vi "Parse Cal String.vi"(3 "error in (no error)":errorcluster={"status"=FALSE, "code"=1073676294, "source"="VISA Read in Read Cal Response.vi"}, 5 "read buffer in":string="19:30:28 105, -1, 1.955 1.954 1.95565 1.954") -> (0 "error out":errorcluster={"status"=FALSE, "code"=1073676294, "source"="VISA Read in Read Cal Response.vi"}, 1 "Cal Data":T1={"Time"="19:30:28", "Consecutive good readings"=105, "Total good readings"=-1, "A/D counts Sensor 1"=1.955, "A/D counts Sensor 2"=1.954, "Diff current/previous Sensor 1"=1.95565, "Diff current/previous Sensor 2"=1.954}, 2 "CAL Complete":bool=TRUE)   [LabVIEW 2013]
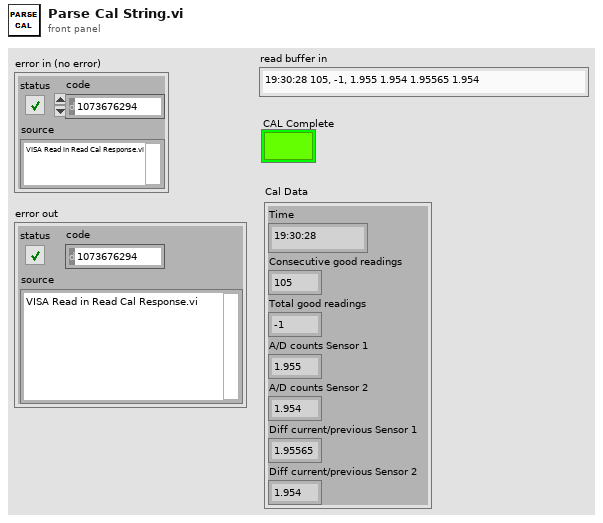
[diagram p1: front panel]
types:
  T1 = cluster{"Time":string, "Consecutive good readings":i32, "Total good readings":i32, "A/D counts Sensor 1":sgl, "A/D counts Sensor 2":sgl, "Diff current/previous Sensor 1":sgl, "Diff current/previous Sensor 2":sgl}
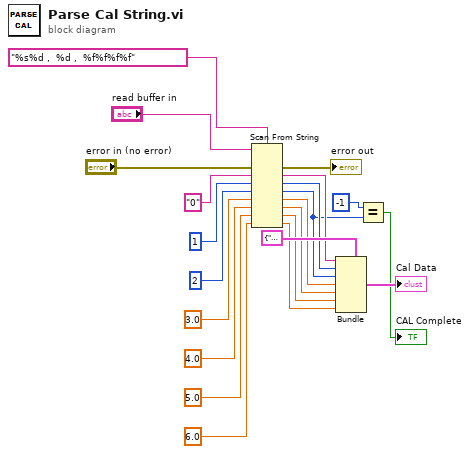
[diagram p0: block diagram]
diagram:
  n1 = Scan From String(format string="%s%d ,  %d ,  %f%f%f%f", input string="read buffer in", error in="error in (no error)", default 1="0" ("default value 1"), default 2=1 ("default value 2"), default 3=2 ("default value 3"), default 4=sgl 3.0 ("default value 7"), default 5=sgl 4.0 ("default value 7"), default 6=sgl 5.0 ("default value 7"), default 7=sgl 6.0 ("default value 7")) -> (error out=→"error out":errorcluster, output 1=w9:string, output 2=w8:i32, output 3=w3:i32, output 4=w7:sgl, output 5=w6:sgl, output 6=w5:sgl, output 7=w4:sgl)  [unwired: 1 in, 2 out]
  n2 = Bundle(cluster=T1 {"Time"="19:30:28", "Consecutive good readings"=105, "Total good readings"=1, "A/D counts Sensor 1"=1.955, "A/D counts Sensor 2"=1.954, "Diff current/previous Sensor 1"=1.95565, "Diff current/previous Sensor 2"=1.954} ("Cal Data"), "Time"=w9, "Consecutive good readings"=w8, "Total good readings"=w3, "A/D counts Sensor 1"=w7, "A/D counts Sensor 2"=w6, "Diff current/previous Sensor 1"=w5, "Diff current/previous Sensor 2"=w4) -> (→"Cal Data":T1)
  n3 = Equal?(x=-1, y=w3) -> (x = y?=→"CAL Complete":bool)
